vi "MCB2400 PWM DBL PrjAttrValidator.vi"(5 "Attr Refnum":refnum<vi>, 9 "PWMNum (0-11)":u8(ring) items=["137", "138", "139", "140", "141", "142"], 11 "Attributes":T1={"Offset%"=50, "Polarity"=FALSE, "Frequency (Hz)"=1000, "Programmable Pin Connections"=0} {"Programmable Pin Connections" items=["PWM0_2_DBL uses the same resources as PWM0_1, PWM0_2, and P3.17. You must remove this EIO from the project if you wish to use any of the other EIO.", "PWM0_4_DBL uses the same resources as PWM0_3, PWM0_4, and P3.19. You must remove this EIO from the project if you wish to use any of the other EIO.", "PWM0_6_DBL uses the same resources as PWM0_5, PWM0_6, and P3.21. You must remove this EIO from the project if you wish to use any of the other EIO.", "PWM1_2_DBL uses the same resources as PWM1_1, PWM1_2, and P2.1. You must remove this EIO from the project if you wish to use any of the other EIO.", "PWM1_4_DBL uses the same resources as PWM1_3, PWM1_4, and P2.4. You must remove this EIO from the project if you wish to use any of the other EIO.", "PWM1_6_DBL uses the same resources as PWM1_5, PWM1_6, and P2.6. You must remove this EIO from the project if you wish to use any of the other EIO."]}) -> (3 "Valid?":bool)   [LabVIEW 2011]
uses:
  <vilib>/Embedded/ARM/MCB2400/MCB2400_PWM_DBL_PrjAttr.ctl
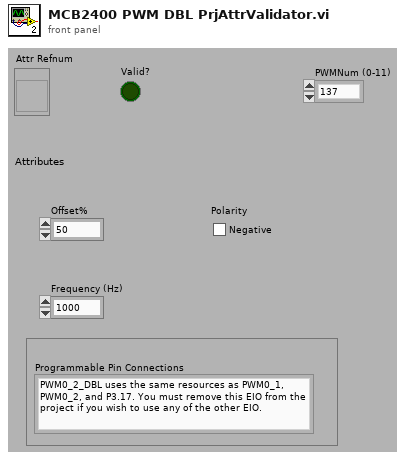
[diagram p1: front panel]
types:
  T1 = typedef "MCB2400_PWM_DBL_PrjAttr.ctl" = cluster{"Offset%":u8, "Polarity":bool, "Frequency (Hz)":u32, "Programmable Pin Connections":u16}
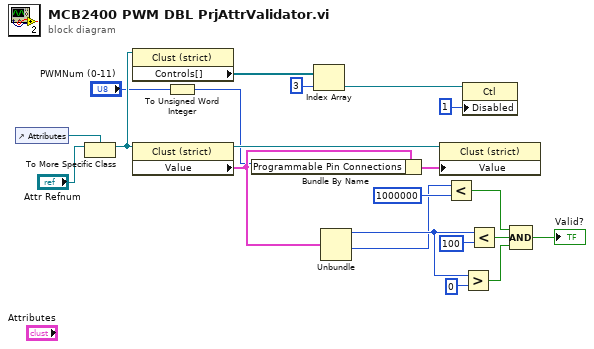
[diagram p0: block diagram]
diagram:
  n1 = control-ref of="Attributes"() -> (w3:refnum<vi>)
  n2 = To More Specific Class(target class=w3, reference="Attr Refnum") -> (specific class reference=w17:refnum<vi>)  [unwired: 1 in, 1 out]
  n3 = property class="Clust (strict)"(reference=w17) -> ("Controls[]"=w14:refnum<vi>[])  [unwired: 1 in, 2 out]
  n4 = property class="Clust (strict)"(reference=w17) -> (reference out=w10:refnum<vi>, "Value"=w9:T1)  [unwired: 1 in, 1 out]
  n5 = To Unsigned Word Integer(number="PWMNum (0-11)") -> (unsigned 16bit integer=w8:u16)
  n6 = Bundle By Name(cluster=w9, "Programmable Pin Connections"=w8) -> (w16:T1)
  n7 = Index Array(array=w14, index=3) -> (element=w19:refnum<vi>)
  n8 = Unbundle(w9) -> ("Offset%"=w5:u8, "Frequency (Hz)"=w4:u32)  [unwired: 2 out]
  n9 = property class="Clust (strict)"(reference=w10, "Value"=w16) -> ()  [unwired: 1 in, 2 out]
  n10 = Less?(x=w4, y=u32 1000000 ("upper limit")) -> (x < y?=w7:bool)
  n11 = property class="Ctl"(reference=w19, "Disabled"=u8 1) -> ()  [unwired: 1 in, 2 out]
  n12 = Greater?(x=w5, y=u8 0 ("lower limit")) -> (0:w1:bool)
  n13 = Less?(x=w5, y=u8 100 ("upper limit")) -> (x < y?=w2:bool)
  n14 = Compound Arithmetic op=AND(w7, w2, w1) -> (→"Valid?":bool)
